vi "Fdx Create UDP Port (TX-CommPort).vi"(6 "VlTx":T1={"domainID"=0, "sideID"=0, "locationID"=0, "interfaceID"=1}, 8 "error in":errorcluster, 9 "VlId":u16, 10 "CommPort Config":T3={"PortType"=enum."FDX_UDP_SAMPLING", "partitionID"=1, "SubVlId"=1, "UdpSrcPort"=1, "UdpDstPort"=1, "SampleRateMs"=128.0, "UdpNumBufMessages"=0, "UdpMaxMessageSize"=1000}, 11 "port handle in":u32) -> (0 "error out":errorcluster, 1 "computedAddresses":T2 {"MACsrc" format="%.0x"}, 2 "commPort handle out":u32, 3 "port handle out":u32)   [LabVIEW 2020, in "AIM664LV.lvlib"]
doc: "This function is used to create a port to transmit data from a specified UDP connection oriented port. Default settings after creation of the UDP port are:\n- UDP port enabled\n- Error injection: OFF\n- Skew (redundand mode only): 0 usec.\nTo change the settings of the UDP port the function FdxCmdTxUDPControl can be used. This function can be used only if transmitter is not running."
uses:
  AIM664LV.lvlib
  _controls/comm_udp_tx.ctl
  _controls/comm_computedMAC-IP.ctl
  helpers/EthFrameManagement/controls/mac_src_info_afdx.ctl
  helpers/EthFrameManagement/controls/ip_src_info_afdx.ctl
  helpers/EthFrameManagement/EthFrameManagement.lvlib
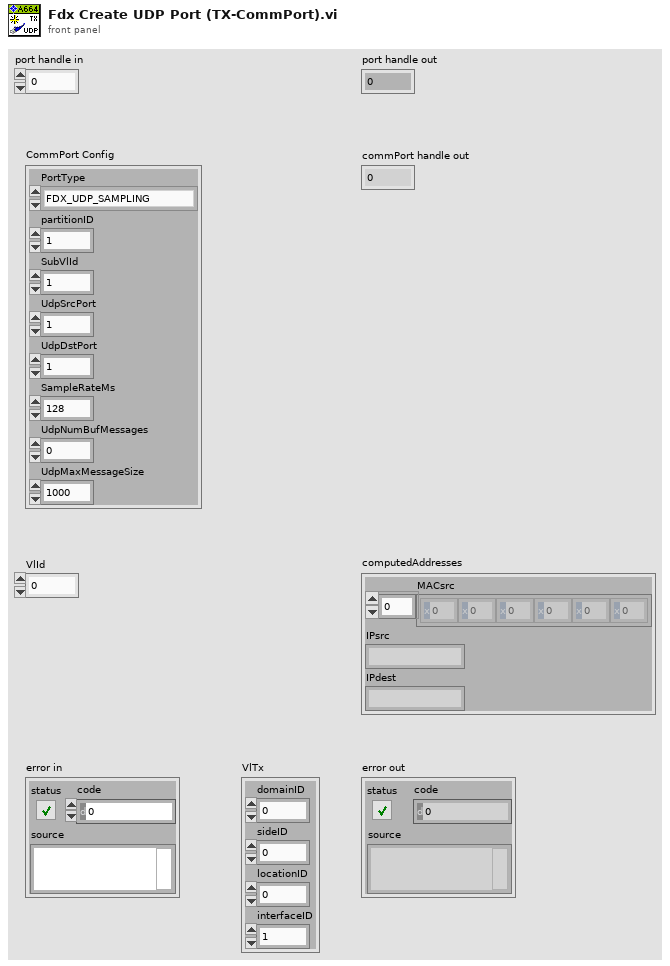
[diagram p1: front panel]
types:
  T1 = typedef "EthFrameManagement.lvlib/mac_src_info_afdx.ctl" = cluster{"domainID":u8, "sideID":u8, "locationID":u8, "interfaceID":u8}
  T2 = typedef "AIM664LV.lvlib/comm_computedMAC-IP.ctl" = cluster{"MACsrc":u8[], "IPsrc":string, "IPdest":string}
  T3 = typedef "AIM664LV.lvlib/comm_udp_tx.ctl" = cluster{"PortType":enum16{"FDX_UDP_SAMPLING", "FDX_UDP_QUEUING"}, "partitionID":u8, "SubVlId":u8, "UdpSrcPort":u16, "UdpDstPort":u16, "SampleRateMs":dbl, "UdpNumBufMessages":u32, "UdpMaxMessageSize":u32}
  T4 = typedef "EthFrameManagement.lvlib/ip_src_info_afdx.ctl" = cluster{"domainID":u8, "sideID":u8, "locationID":u8, "partitionID":u8}
  T5 = cluster{"PortType":u32, "UdpSrc":u32, "IpSrc":u32, "VlId":u32, "IpDst":u32, "UdpDst":u32, "SubVlId":u32, "UdpNumBufMessages":u32, "UdpMaxMessageSize":u32, "UdpSamplingRate":u32}
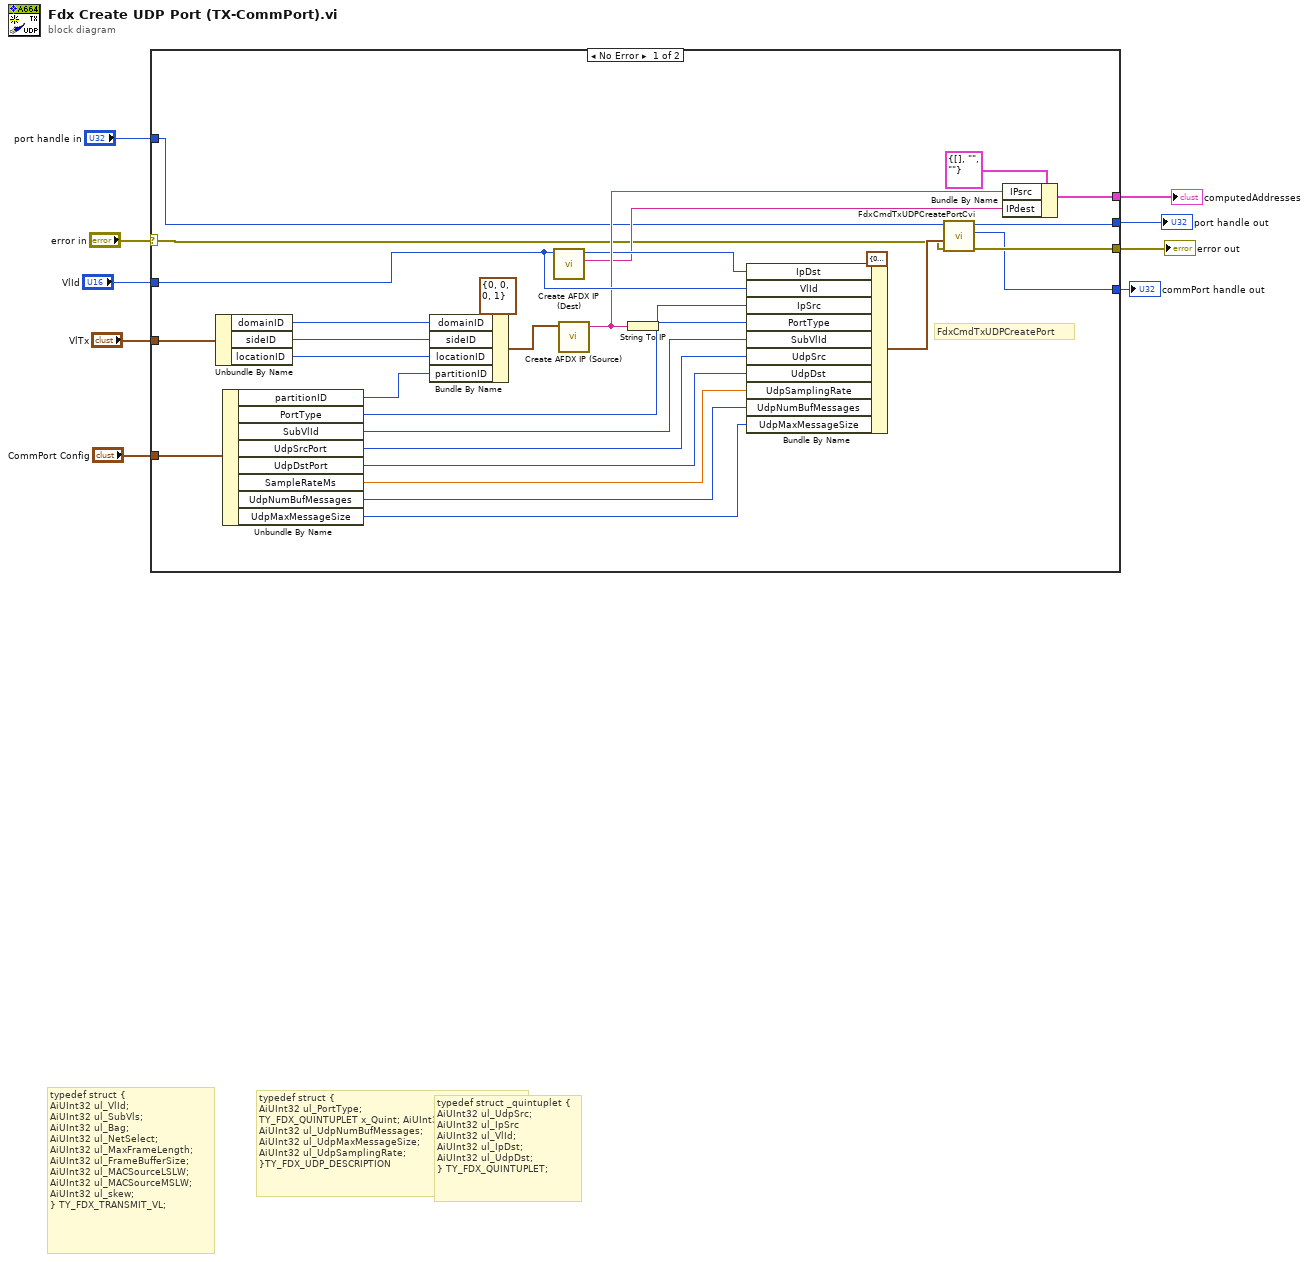
[diagram p0: block diagram]
diagram:
  # "typedef struct _quintuplet {\nAiUInt32 ul_UdpSrc;\nAiUInt32 ul_IpSrc\nAiUInt32 ul_VlId;\nAiUInt32 ul_IpDst;\nAiUInt32 ul_UdpDst;\n} TY_FDX_QUINTUPLET;"
  # "typedef struct {\nAiUInt32 ul_PortType;\nTY_FDX_QUINTUPLET x_Quint; AiUInt32 ul_SubVlId;\nAiUInt32 ul_UdpNumBufMessages;\nAiUInt32 ul_UdpMaxMessageSize;\nAiUInt32 ul_UdpSamplingRate;\n}TY_FDX_UDP_DESCRIPTION"
  # "typedef struct {\nAiUInt32 ul_VlId;\nAiUInt32 ul_SubVls;\nAiUInt32 ul_Bag;\nAiUInt32 ul_NetSelect;\nAiUInt32 ul_MaxFrameLength;\nAiUInt32 ul_FrameBufferSize;\nAiUInt32 ul_MACSourceLSLW;\nAiUInt32 ul_MACSourceMSLW;\nAiUInt32 ul_skew;\n} TY_FDX_TRANSMIT_VL;"
  n1 = case shown="No Error" "error in" {
    selector: "error in" -> [w12 w39]
    tunnel: "port handle in" -> [w13 w40]
    tunnel: [w11 w40] -> w7
    tunnel: [w37 w39] -> w6
    tunnel: "CommPort Config" -> [w38 _]
    tunnel: [w36 _] -> w4
    tunnel: "VlId" -> [w35 _]
    tunnel: "VlTx" -> [w14 _]
    tunnel: [w10 _] -> w1
    frame No Error {
      # "FdxCmdTxUDPCreatePort"
      n2 = Unbundle By Name(w14) -> ("domainID"=w17:u8, "sideID"=w16:u8, "locationID"=w15:u8)
      n3 = Unbundle By Name(w38) -> ("partitionID"=w27:u8, "PortType"=w25:enum16{"FDX_UDP_SAMPLING", "FDX_UDP_QUEUING"}, "SubVlId"=w24:u8, "UdpSrcPort"=w23:u16, "UdpDstPort"=w22:u16, "SampleRateMs"=w21:dbl, "UdpNumBufMessages"=w20:u32, "UdpMaxMessageSize"=w19:u32)
      n4 = Bundle By Name(cluster=T4 {"domainID"=0, "sideID"=0, "locationID"=0, "partitionID"=1} ("Source Info"), "domainID"=w17, "sideID"=w16, "locationID"=w15, "partitionID"=w27) -> (w31:T4)
      n5 = call "Create AFDX IP (Dest).vi"("VL"=w35) -> ("ip string"=w18:string, "ip net"=w28:u32)  [unwired: 9 in]
      n6 = call "Create AFDX IP (Source).vi"("Source Info"=w31) -> ("ip address"=w29:string)  [unwired: 10 in]
      n7 = String To IP(1:w29) -> (0:w26:u32)
      n8 = Bundle By Name(cluster=T5 {"PortType"=0, "UdpSrc"=0, "IpSrc"=0, "VlId"=0, "IpDst"=0, "UdpDst"=0, "SubVlId"=0, "UdpNumBufMessages"=0, "UdpMaxMessageSize"=0, "UdpSamplingRate"=0} ("UdpDescription"), "IpDst"=w28, "VlId"=w35, "IpSrc"=w26, "PortType"=w25, "SubVlId"=w24, "UdpSrc"=w23, "UdpDst"=w22, "UdpSamplingRate"=w21, "UdpNumBufMessages"=w20, "UdpMaxMessageSize"=w19) -> (w33:T5)
      n9 = call "FdxCmdTxUDPCreatePortCvi.vi"("error in"=w12, "UdpDescription"=w33, "InstrumentHandle"=w13) -> ("error out"=w37:errorcluster, "UdpHandle"=w10:u32, "InstrumentHandle"=w11:u32)  [unwired: 6 in]
      n10 = Bundle By Name(cluster=T2 {"MACsrc"=[], "IPsrc"="", "IPdest"=""} ("computedAddresses"), "IPsrc"=w29, "IPdest"=w18) -> (w36:T2)
    }
    frame Error {
    }
  }
  "port handle out" <- w7
  "error out" <- w6
  "computedAddresses" <- w4
  "commPort handle out" <- w1
